vi "Sort (single).vi"(8 "error in (no error)":errorcluster, 9 "Use Sort Pointers (F)":bool, 10 "Sort Pointers":i32[](array[numeric]), 11 "XY-data":cluster{"X-array":dbl[], "Y-array":dbl[]}) -> (0 "error out":errorcluster, 2 "Sorted Pointers":i32[](array[numeric]), 3 "Sorted XY-data out":cluster{"X-array":dbl[], "Y-array":dbl[]} {"Y-array" format="%.2p"; "X-array" format="%.2p"})   [LabVIEW 2019, in "xy_utilities.lvlib"]
doc: "Sorts the input <b>XY-data</b> according to its x array.\n\nIf <b>Use Sort Pointers</b> = <b>True</b> then sort according to <b>Sort Pointers</b>.\n\nWire data to the data input to determine the polymorphic instance to use or manually select the instance."
uses:
  xy_utilities.lvlib
  <userlib>/_OpenG.lib/array/array.llb/Sort 1D Array (DBL)__ogtk.vi
  <userlib>/_OpenG.lib/array/array.llb/Reorder 1D Array2 (DBL)__ogtk.vi
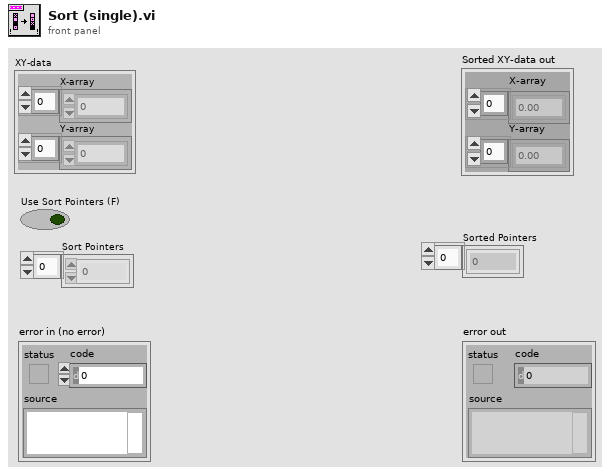
[diagram p1: front panel]
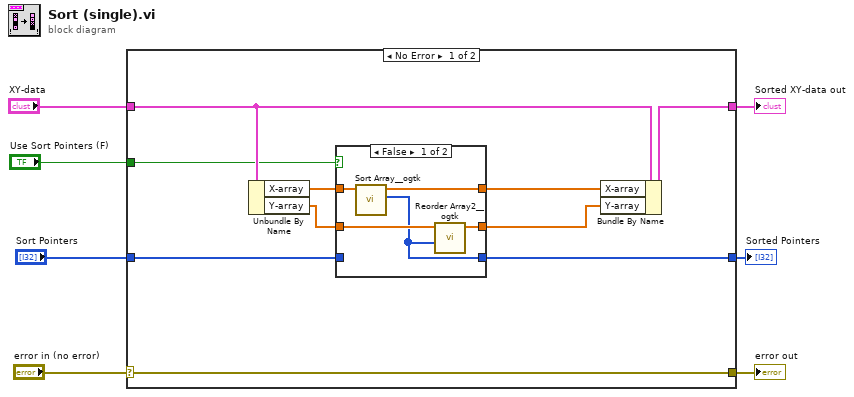
[diagram p0: block diagram]
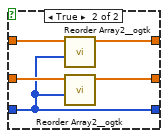
[diagram p2: hidden frame]
diagram:
  n1 = case shown="No Error" "error in (no error)" {
    selector: "error in (no error)" -> [w17 w30]
    tunnel: [w17 w30] -> w6
    tunnel: "XY-data" -> [w16 w29]
    tunnel: [w15 w29] -> w4
    tunnel: [w10 w28] -> w3
    tunnel: "Sort Pointers" -> [w9 w28]
    tunnel: "Use Sort Pointers (F)" -> [w8 _]
    frame No Error {
      n2 = Unbundle By Name(w16) -> ("X-array"=w14:dbl[], "Y-array"=w13:dbl[])
      n3 = case shown="False" w8 {
        tunnel: w14 -> [w22 w27]
        tunnel: w13 -> [w21 w25]
        tunnel: [w20 w26] -> w12
        tunnel: [w19 w24] -> w11
        tunnel: [w18 w23] -> w10
        tunnel: w9 -> [_ w23]
        frame False {
          n4 = call-poly <userlib>:"Sort Array__ogtk.vi"("Array in"=w22) -> ("Sorted Pointers"=w18:i32[], "Sorted Array out"=w20:dbl[])  [unwired: 9 in]
          n5 = call-poly <userlib>:"Reorder Array2__ogtk.vi"("indices"=w18, "array"=w21) -> ("reordered array"=w19:dbl[])  [unwired: 9 in]
        }
        frame True {
          n6 = call-poly <userlib>:"Reorder Array2__ogtk.vi"("indices"=w23, "array"=w27) -> ("reordered array"=w26:dbl[])  [unwired: 9 in]
          n7 = call-poly <userlib>:"Reorder Array2__ogtk.vi"("indices"=w23, "array"=w25) -> ("reordered array"=w24:dbl[])  [unwired: 9 in]
        }
      }
      n8 = Bundle By Name(cluster=w16, "X-array"=w12, "Y-array"=w11) -> (w15:cluster{"X-array":dbl[], "Y-array":dbl[]})
    }
    frame Error {
    }
  }
  "error out" <- w6
  "Sorted XY-data out" <- w4
  "Sorted Pointers" <- w3
